vi "Programa_Ppal.vi"() -> ()   [LabVIEW 2019]
uses:
  <vilib>/addons/Control Design/_Model Construction/Model Creation.llb/Model Creation SubVI/cd_Create Transfer Function Model.vi
  <vilib>/addons/Control Design/_Utility/Model Viewer.llb/Model Viewer SubVI/cd_Draw Transfer Function Equation (TF).vi
  <vilib>/functionblocks/Control/PID/PID.vi
  <vilib>/functionblocks/FB Core/FB Core.xnode
  <vilib>/addons/Control Design/_Model Construction/NI_LinSys_Model Creation.lvlib
  <vilib>/addons/Control Design/_Utility/NI_CD_Model Viewer.lvlib
  <vilib>/functionblocks/NI_FunctionBlock Libraries.lvlib
panel:
  in  "?":enum32{"Lazo Abierto", "Lazo de control"}(radio)
  out "Función de Transferencia":picture
  in  "RETARDO FT":dbl
  in  "SET-POINT (%)":dbl=25.0
  in  "stop":bool
  out "RESPUESTA PLANTA":dbl=12.500000564078626 format="%.2f"
  out "?":T1(graph)={"Set-point (%)"=25.0, "Y% esc y filt"=25.0, "Ley uk"=12.500000564078626}
  in  "NUMERADOR FT":dbl[](array[numeric])=[1.0, 1.0]
  in  "DENOMINADOR FT":dbl[](array[numeric])=[1.0, 1.0, 2.0]
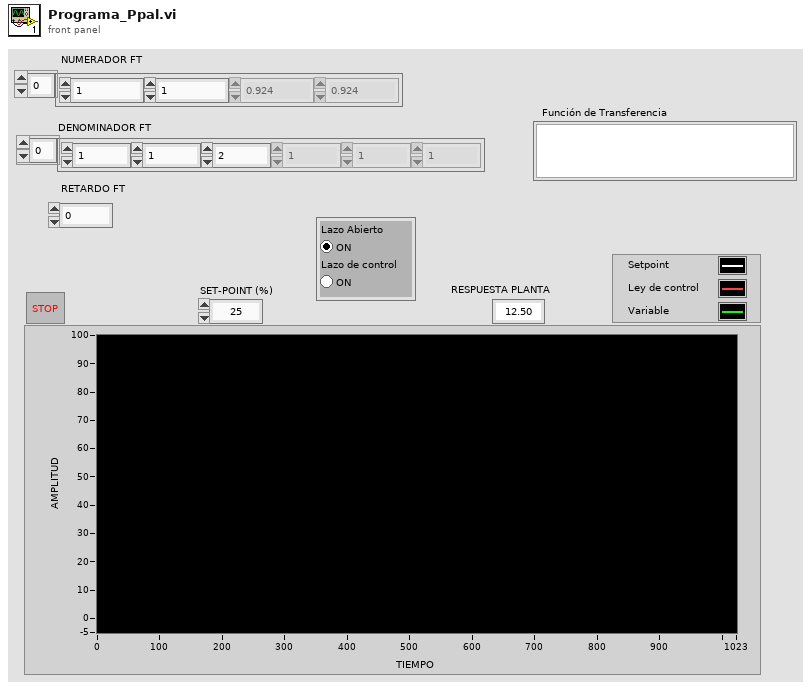
[diagram p1: front panel]
types:
  T1 = cluster{"Set-point (%)":dbl, "Y% esc y filt":dbl, "Ley uk":dbl}
  T2 = cluster{"Set-point (%)":dbl, "Y% esc y filt":dbl, "Ley uk":dbl}[]
  T3 = typedef "NI_Matrix.lvlib/RealMatrix.ctl" = dbl[][]
  T4 = cluster{"SET-POINT (%)":dbl, "output":dbl, "Y(kt)":dbl}
  T5 = typedef "NI_LinSys_Model Typedefs.lvlib/CD Transfer Function Model (MIMO).ctl" = cluster{"properties":T6, "transfer function(s)":T7[][]}
  T6 = typedef "NI_LinSys_Model Typedefs.lvlib/CD General Elements.ctl" = cluster{"Model name":string, "Input names":string[], "Output names":string[], "Input Delays":dbl[], "Output Delays":dbl[], "Sampling Time":dbl, "Notes":string}
  T7 = typedef "NI_LinSys_Model Typedefs.lvlib/CD Transfer Function Model (SISO).ctl" = cluster{"Numerator":dbl[], "Denominator":dbl[], "delay":dbl}
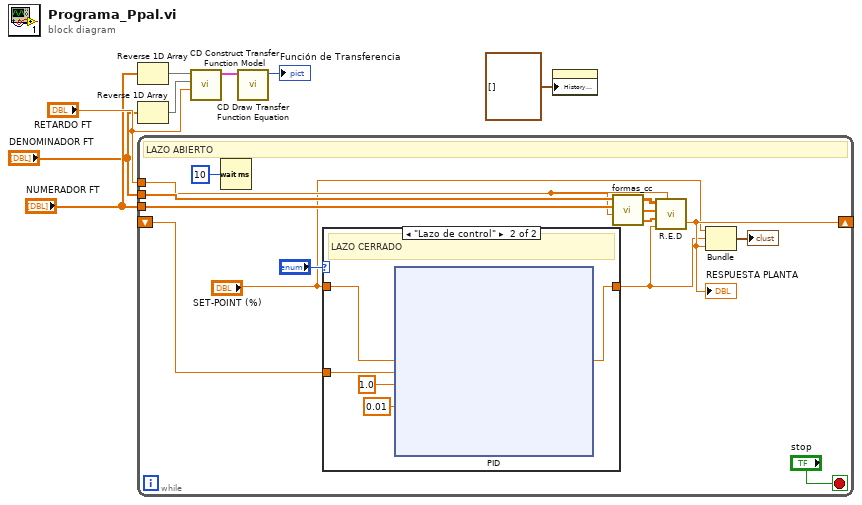
[diagram p0: block diagram]
diagram:
  n1 = Reverse 1D Array(array="NUMERADOR FT") -> (reversed array=w3:dbl[])
  n2 = Reverse 1D Array(array="DENOMINADOR FT") -> (reversed array=w2:dbl[])
  n3 = while {
    tunnel: "DENOMINADOR FT" -> [w19]
    tunnel: "NUMERADOR FT" -> [w18]
    tunnel: "RETARDO FT" -> [w15]
    shift-right: [w14] -> _
    shift-left: _ -> [w13]
    stop <- "stop" stop-if-true
    # "LAZO ABIERTO"
    n4 = Wait (ms)(milliseconds to wait=u32 10) -> ()  [unwired: 1 out]
    n5 = case shown="\"Lazo de control\"" "?" {
      tunnel: "SET-POINT (%)" -> [w23 w28]
      tunnel: w13 -> [_ w27]
      tunnel: [w23 w26] -> w12
      frame "Lazo Abierto", Default {
      }
      frame "Lazo de control" {
        # "LAZO CERRADO"
        n6 = xnode "PID"("setpoint"=w28, "process variable"=w27, "proportional gain (Kc)"=1.0, "integral time (Ti, min)"=0.01) -> ("output"=w26:dbl)  [unwired: 3 in, 1 out]
      }
    }
    n7 = call "formas_cc.vi"("retardo"=w15, "Numerador"=w18, "Denominador"=w19) -> ("Vector C"=w20:dbl[], "Vector B"=w21:dbl[], "Matriz A"=w22:T3)  [unwired: 1 in]
    n8 = call "R.E.D.vi"("A"=w22, "B"=w21, "C"=w20, "u(k)"=w12, "Retardo"=w15) -> ("Y(kt)"=w14:dbl)  [unwired: 1 out]
    "RESPUESTA PLANTA" <- w14
    n9 = Bundle("SET-POINT (%)"="SET-POINT (%)", "output"=w12, "Y(kt)"=w14) -> (→"?":T4)  [unwired: 1 in]
  }
  n10 = call-poly <vilib>:"CD Construct Transfer Function Model.vi"("Delay"="RETARDO FT", "Denominator"=w2, "Numerator"=w3) -> ("Transfer Function Model"=w1:T5)  [unwired: 7 in, 1 out]
  n11 = call-poly <vilib>:"CD Draw Transfer Function Equation.vi"("Transfer Function Model"=w1) -> ("Equation"=→"Función de Transferencia":picture)  [unwired: 8 in, 2 out]
  n12 = property class="WFChart (strict)"("History Data"=T2 []) -> ()  [unwired: 2 in, 2 out]
